vi "ECG_MAIN VI.vi"() -> ()   [LabVIEW 2021]
uses:
  <vilib>/express/express analysis/Spectral/Block/exnSpectralBlock spectral measurements peak poly.vi
  <vilib>/express/express analysis/Spectral/Block/exnSpectralBlock spectral measurements peak WFM.vi
  <vilib>/express/express analysis/Spectral/XNode/ExpressSpectralMeasurementsBlockNode.xnode
  <vilib>/Analysis/NI_AALBase.lvlib
panel:
  in  "SHUTDOWN":bool
  out "RR Interval":dbl[](graph)
  out "Heart Beat":dbl[](graph)
  out "Phase":cluster{"f0":dbl, "df":dbl, "magnitude":dbl[]}(graph)
  out "Magnitude":cluster{"f0":dbl, "df":dbl, "magnitude":dbl[]}(graph)
  out "Filtered ECG Signal":waveform(dbl)[](graph)
  out "Heart Rate":dbl
  out "Histogram Graph":T1(graph)
  out "ECG sample":waveform(dbl)(graph)
  out "Raw ECG signal":waveform(dbl)(graph)
  # "EEG SIGNAL FILTERING AND PARAMETERS EXTRACTION"
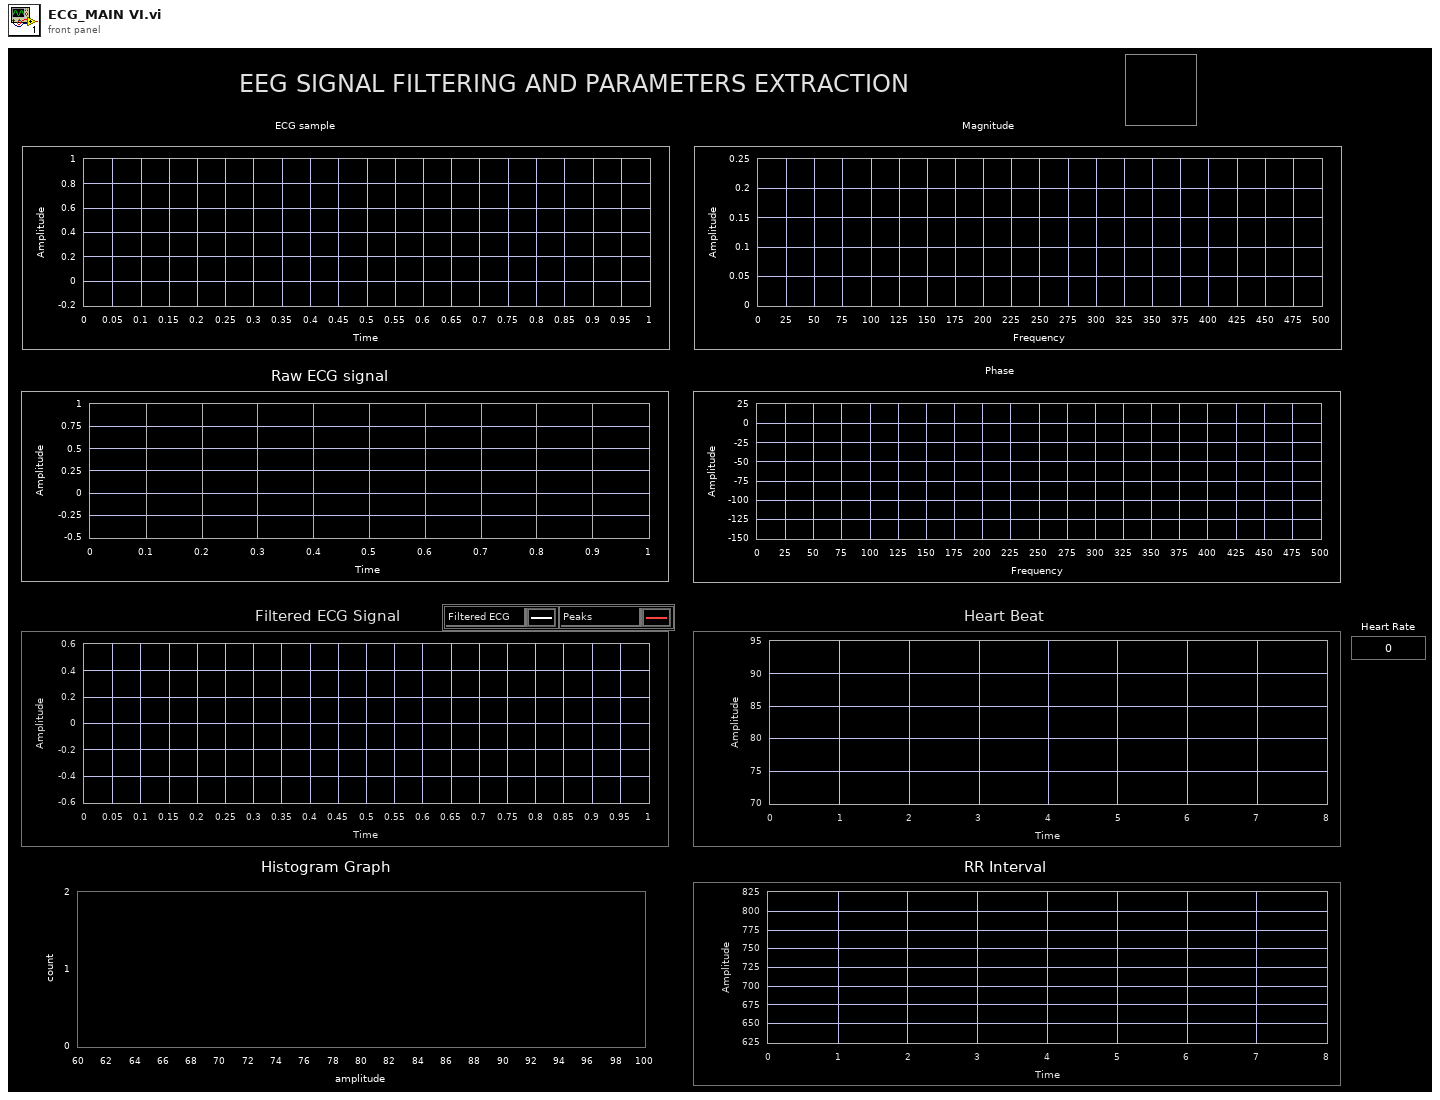
[diagram p1: front panel]
types:
  T1 = cluster{"X Values":dbl[], "Histogram: h(x)":i32[]}
  T2 = cluster{"averaging mode":u16, "weighting mode":u16, "number of averages":u32}
  T3 = cluster{"dB On (F)":bool, "unwrap phase (F)":bool, "convert to degree (F)":bool}
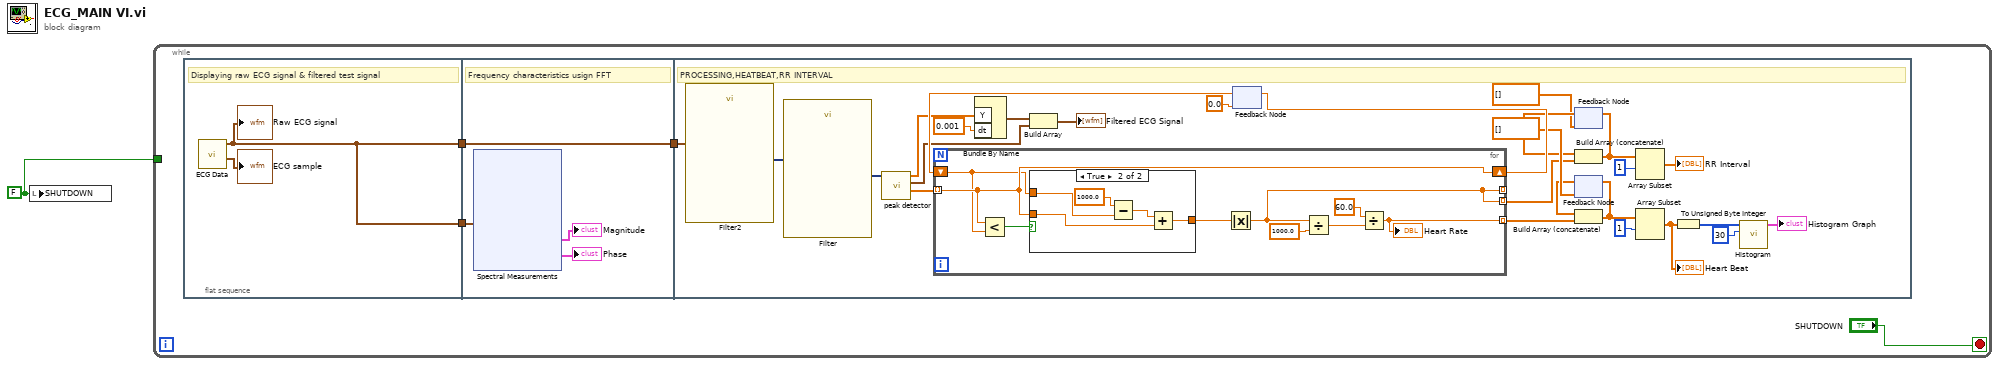
[diagram p0: block diagram]
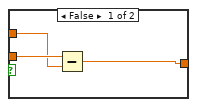
[diagram p2: hidden frame]
diagram:
  w1 = FALSE ("SHUTDOWN")
  n1 = local write "SHUTDOWN"(w1) -> ()
  n2 = while {
    tunnel: w1 -> [_]
    stop <- "SHUTDOWN" stop-if-true
    n3 = flat-sequence {
      tunnel: [w7] -> w5
      tunnel: [w7] -> w4
      tunnel: w5 -> [w10]
      tunnel: w4 -> [w11]
      tunnel: [w11] -> w3
      tunnel: w3 -> [w31]
      frame #0 {
        # "Displaying raw ECG signal & filtered test signal"
        n4 = call "ECG Data.vi"() -> ("Clean ECG"=→"ECG sample":waveform(dbl), "Noisy ECG"=w7:waveform(dbl))  [unwired: 10 in]
        "Raw ECG signal" <- w7
      }
      frame #1 {
        # "Frequency characteristics usign FFT"
        n5 = xnode "Spectral Measurements"("Signals"=w10) -> ("FFT - (Peak)"=→"Magnitude":cluster{"f0":dbl, "df":dbl, "magnitude":dbl[]}, "Phase"=→"Phase":cluster{"f0":dbl, "df":dbl, "phase":dbl[]})  [unwired: 1 in, 1 out]
      }
      frame #2 {
        # "PROCESSING,HEATBEAT,RR INTERVAL"
        n6 = call "Filter2"("Signal"=w31) -> ("Filtered Signal"=w48:dynamicdata)  [unwired: 9 in, 1 out]
        n7 = call "Filter"("Signal"=w48) -> ("Filtered Signal"=w32:dynamicdata)  [unwired: 9 in, 1 out]
        n8 = call "peak detector.vi"("Filtered Signal"=w32) -> ("Locations"=w47:dbl[], "Waveform"=w35:waveform(dbl), "Y"=w37:dbl[])  [unwired: 8 in]
        n9 = Bundle By Name("Y"=w37, "dt"=0.001) -> (w36:waveform(dbl))  [unwired: 1 in]
        n10 = Build Array(w36, w35) -> (→"Filtered ECG Signal":waveform(dbl)[])
        n11 = feedback #1(0.0) -> (w44:dbl)
        n12 = for {
          tunnel: w47 -> [w54] mode=indexing
          tunnel: [w50] -> w46 mode=indexing
          shift-right: [w54] -> w45
          shift-left: w44 -> [w52]
          tunnel: [w49] -> _ mode=indexing
          tunnel: [w49] -> w26 mode=indexing
          n13 = Less?(x=w54, y=w52) -> (x < y?=w53:bool)
          n14 = case shown="True" w53 {
            tunnel: w54 -> [w60 w61]
            tunnel: w52 -> [w59 w62]
            tunnel: [w58 w63] -> w51
            frame False {
              n15 = Subtract(x=w60, y=w59) -> (x-y=w58:dbl)
            }
            frame True {
              n16 = Subtract(x=1000.0, y=w62) -> (x-y=w64:dbl)
              n17 = Add(x=w64, y=w61) -> (x+y=w63:dbl)
            }
          }
          n18 = Absolute Value(x=w51) -> (abs(x)=w49:dbl)
          n19 = Divide(x=w49, y=1000.0) -> (x/y=w55:dbl)
          n20 = Divide(x=60.0, y=w55) -> (x/y=w50:dbl)
          "Heart Rate" <- w50
        }
        n21 = feedback-in #1(w45) -> ()
        n22 = feedback #2(dbl[] []) -> (w27:dbl[])
        n23 = Build Array (concatenate)(w27, w26) -> (w25:dbl[])
        n24 = feedback-in #2(w25) -> ()
        n25 = feedback #3(dbl[] []) -> (w30:dbl[])
        n26 = Build Array (concatenate)(w30, w46) -> (w28:dbl[])
        n27 = feedback-in #3(w28) -> ()
        n28 = Array Subset(array=w25, index=1) -> (→"RR Interval":dbl[])  [unwired: 1 in]
        n29 = Array Subset(array=w28, index=1) -> (w29:dbl[])  [unwired: 1 in]
        "Heart Beat" <- w29
        n30 = To Unsigned Byte Integer(number=w29) -> (unsigned 8bit integer=w42:u8[])
        n31 = call <vilib>:"Histogram.vi"("intervals"=30, "X"=w42) -> ("Histogram Graph"=→"Histogram Graph":T1)  [unwired: 6 in, 3 out]
      }
    }
  }
